vi "evo irimager get thermal image size.vi"(10 "h":i32, 11 "w":i32) -> (1 "function return":i32, 2 "h out":i32, 3 "w out":i32)   [LabVIEW 2017]
doc: "DIRECT_API int evo_irimager_get_thermal_image_size(int* w, int* h);"
uses:
  libirimager.dll
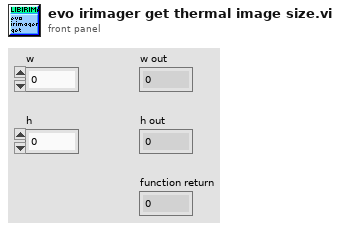
[diagram p1: front panel]
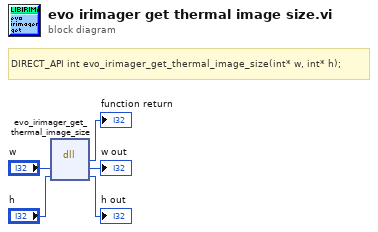
[diagram p0: block diagram]
diagram:
  # "DIRECT_API int evo_irimager_get_thermal_image_size(int* w, int* h);"
  n1 = dll-call lib="C:/Users/evocortex/workspace/irdirectsdk/src/sdk/examples/generic/labview/libirimager.dll" fn="evo_irimager_get_thermal_image_size"("w"="w", "h"="h") -> ("Rückgabetyp"=→"function return":i32, "w"=→"w out":i32, "h"=→"h out":i32)  [unwired: 3 in, 2 out]
